vi "Cost function.vi"(1 "SoC":dbl, 2 "SoC_T":dbl, 3 "Srated":dbl) -> (0 "cost-function":T1)   [LabVIEW 2021]
doc: "This VI computes the Cost Function. It takes as inputs the target state of charge SoCTARGET, the current state of charge SoCt, the active power boundaries (Ptmin, Ptmax), and the constants ab, bb, cb, k presented in equation (23). It returns as outputs the representation of the advertisement message of the Cost Function as a matrix, and a graphical representation of the Cost Function in a Cost/P plane. \n\nThe VI is based on the model presented in this project, taking into consideration equations (23), …, (29)."
uses:
  General purpose/cost-function.ctl
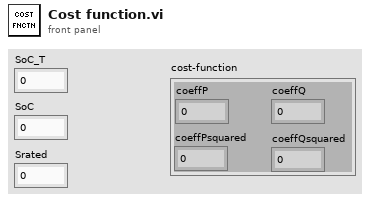
[diagram p1: front panel]
types:
  T1 = typedef "cost-function.ctl" = cluster{"coeffPsquared":dbl, "coeffP":dbl, "coeffQsquared":dbl, "coeffQ":dbl}
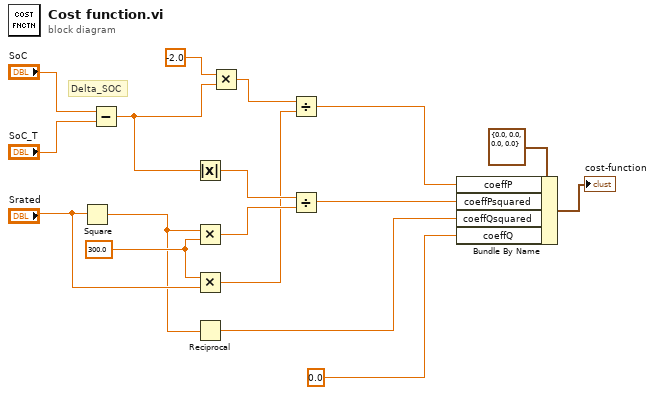
[diagram p0: block diagram]
diagram:
  w13 = 300.0 ("y")
  # "Delta_SOC"
  n1 = Square(x="Srated") -> (x^2=w7:dbl)
  n2 = Subtract(x="SoC", y="SoC_T") -> (x-y=w14:dbl)
  n3 = Absolute Value(x=w14) -> (abs(x)=w11:dbl)
  n4 = Multiply(x=w7, y=w13) -> (x*y=w10:dbl)
  n5 = Multiply(x=w13, y="Srated") -> (x*y=w8:dbl)
  n6 = Reciprocal(x=w7) -> (1/x=w4:dbl)
  n7 = Multiply(x=-2.0, y=w14) -> (x*y=w9:dbl)
  n8 = Divide(x=w9, y=w8) -> (x/y=w2:dbl)
  n9 = Divide(x=w11, y=w10) -> (x/y=w3:dbl)
  n10 = Bundle By Name(cluster=T1 {"coeffPsquared"=0.0, "coeffP"=0.0, "coeffQsquared"=0.0, "coeffQ"=0.0} ("cost-function"), "coeffP"=w2, "coeffPsquared"=w3, "coeffQsquared"=w4, "coeffQ"=0.0) -> (→"cost-function":T1)
